vi "Parse Data to Clusters.vi"(8 "year":i32=1970, 9 "month":i32=1, 10 "day of month":i32=1, 11 "body Text":string) -> (3 "Result Data Array":T1[](array[typedef]))   [LabVIEW 2012]
uses:
  TypeDef/WeatherData.ctl
panel:
  out "Cleaned Text":string
  in  "Col Hedders":string[](array[string])
  out "Body Data":string[][](array[string])
  # "Time"
  # "Float"
  # "Float"
  # "Int"
  # "Float"
  # "Float"
  # "VARCHAR(10)"
  # "Float"
  # "Float"
  # "Float"
  # "VARCHAR(45)"
  # "VARCHAR(45)"
  # "INT"
  # "Date time"
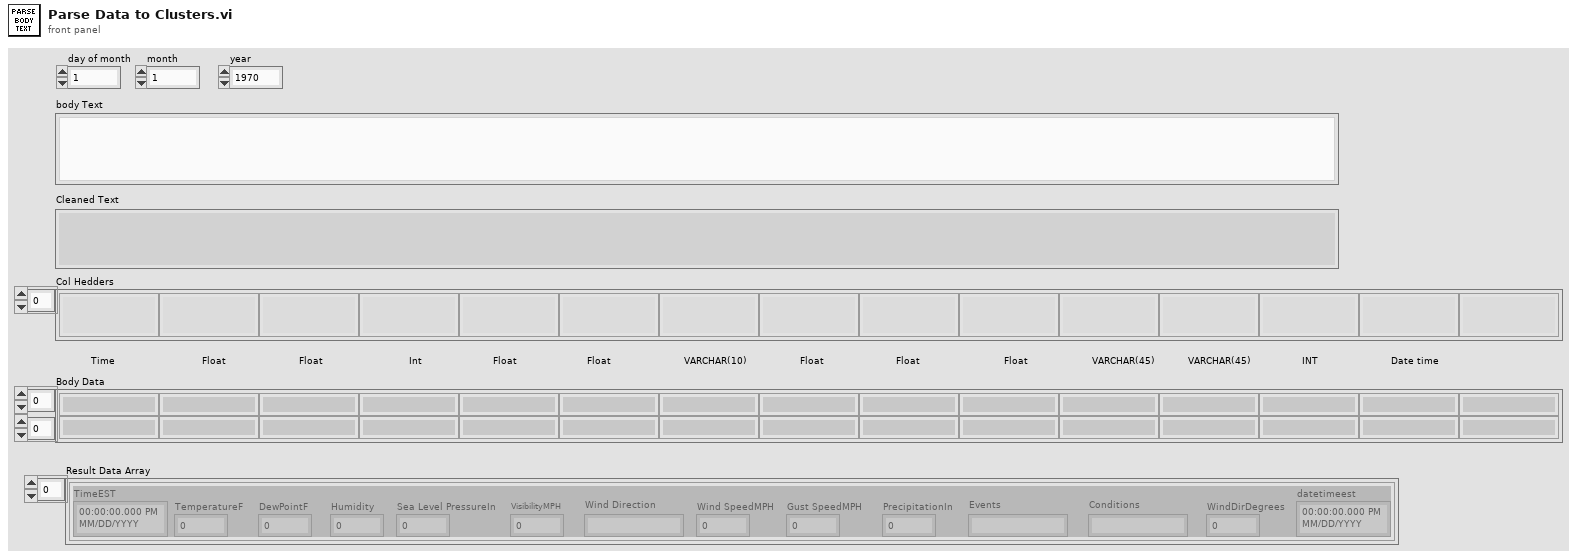
[diagram p1: front panel]
types:
  T1 = typedef "WeatherData.ctl" = cluster{"TimeEST":timestamp, "TemperatureF":dbl, "DewPointF":dbl, "Humidity":i32, "Sea Level PressureIn":dbl, "VisibilityMPH":dbl, "Wind Direction":string, "Wind SpeedMPH":dbl, "Gust SpeedMPH":dbl, "PrecipitationIn":dbl, "Events":string, "Conditions":string, "WindDirDegrees":i32, "datetimeest":timestamp}
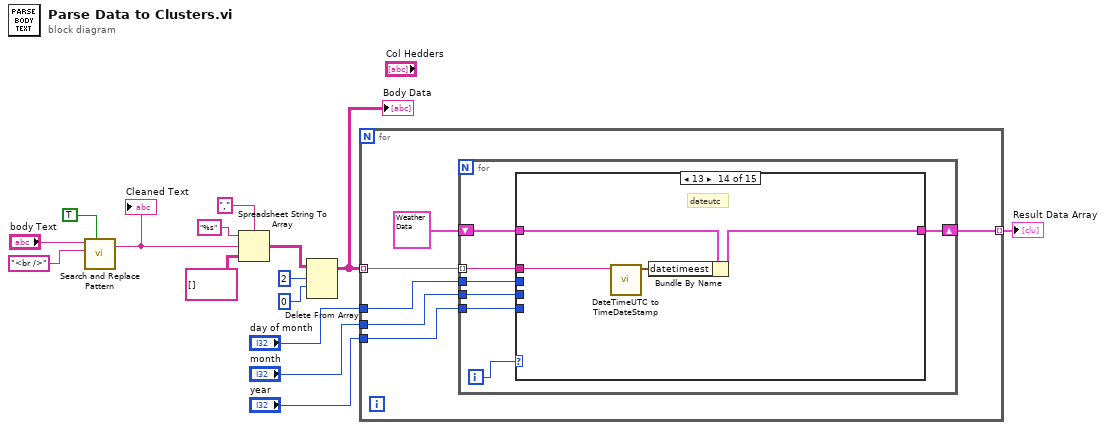
[diagram p0: block diagram]
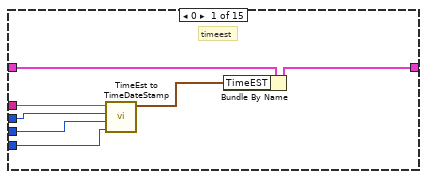
[diagram p2: hidden frame]
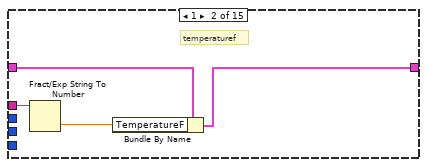
[diagram p3: hidden frame]
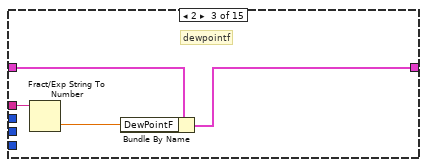
[diagram p4: hidden frame]
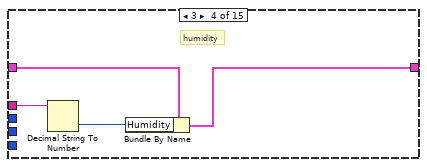
[diagram p5: hidden frame]
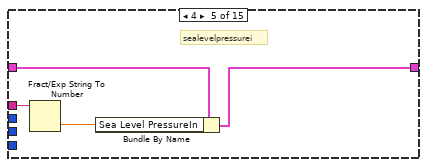
[diagram p6: hidden frame]
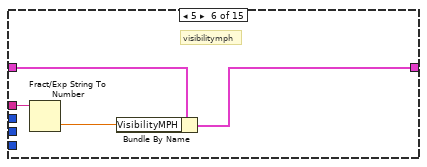
[diagram p7: hidden frame]
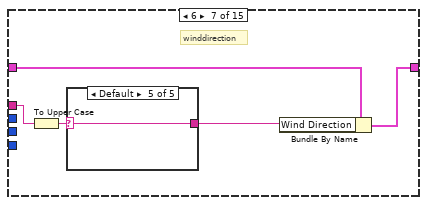
[diagram p8: hidden frame]
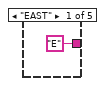
[diagram p9: hidden frame]
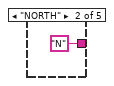
[diagram p10: hidden frame]
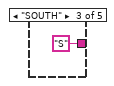
[diagram p11: hidden frame]
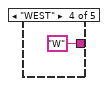
[diagram p12: hidden frame]
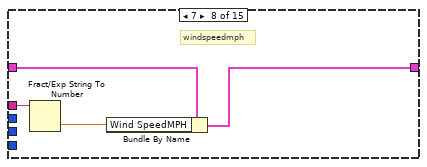
[diagram p13: hidden frame]
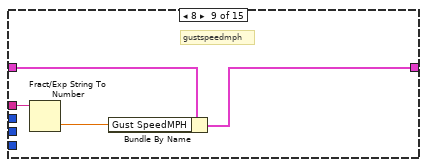
[diagram p14: hidden frame]
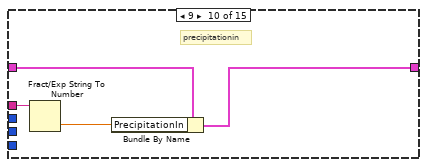
[diagram p15: hidden frame]
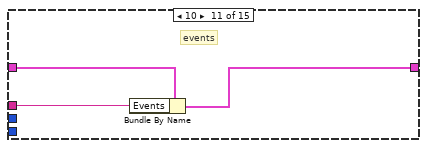
[diagram p16: hidden frame]
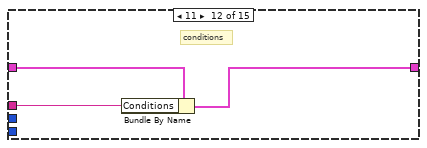
[diagram p17: hidden frame]
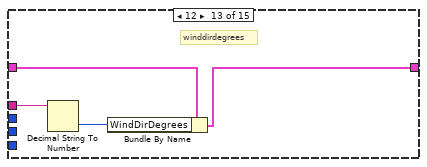
[diagram p18: hidden frame]
diagram:
  n1 = call <vilib>:"Search and Replace Pattern.vi"("string"="body Text", "regular expression (\"\")"="<br />" ("regular expression (\"\")"), "replace all? (F)"=TRUE) -> ("result string"=w6:string)  [unwired: 2 in, 1 out]
  "Cleaned Text" <- w6
  n2 = Spreadsheet String To Array(delimiter (Tab)=",", format string="%s", spreadsheet string=w6, array type (2D Dbl)=string[][] []) -> (array=w12:string[][])
  n3 = Delete From Array(array=w12, length=2, index (row)=0) -> (array with subset deleted=w9:string[][])  [unwired: 1 in, 1 out]
  "Body Data" <- w9
  n4 = for {
    tunnel: w9 -> [w20] mode=indexing
    tunnel: [w19] -> w8 mode=indexing
    tunnel: "day of month" -> [w18]
    tunnel: "month" -> [w17]
    tunnel: "year" -> [w16]
    n5 = for {
      tunnel: w20 -> [w27] mode=indexing
      shift-right: [w25] -> w19
      shift-left: T1 {"TimeEST"=timestamp(0 s since 1904-01-01), "TemperatureF"=0.0, "DewPointF"=0.0, "Humidity"=0, "Sea Level PressureIn"=0.0, "VisibilityMPH"=0.0, "Wind Direction"="", "Wind SpeedMPH"=0.0, "Gust SpeedMPH"=0.0, "PrecipitationIn"=0.0, "Events"="", "Conditions"="", "WindDirDegrees"=0, "datetimeest"=timestamp(0 s since 1904-01-01)} ("weatherdata") -> [w26]
      tunnel: w18 -> [w24]
      tunnel: w17 -> [w23]
      tunnel: w16 -> [w22]
      i -> [w28]
      n6 = case shown="13" w28 {
        tunnel: w27 -> [w33 w39 w43 w45 w51 w55 w58 w69 w73 w77 w78 w81 w85 w89 _]
        tunnel: w26 -> [w35 w37 w41 w47 w49 w53 w60 w67 w71 w75 w80 w83 w87 w91 w92]
        tunnel: [w34 w36 w40 w46 w48 w52 w59 w66 w70 w74 w79 w82 w86 w90 w92] -> w25
        tunnel: w24 -> [w31 _ _ _ _ _ _ _ _ _ _ _ _ _ _]
        tunnel: w23 -> [w30 _ _ _ _ _ _ _ _ _ _ _ _ _ _]
        tunnel: w22 -> [w29 _ _ _ _ _ _ _ _ _ _ _ _ _ _]
        frame 0 {
          # "timeest"
          n7 = call "TimeEst to TimeDateStamp.vi"("year"=w29, "month"=w30, "day of month"=w31, "Time String"=w33) -> ("time stamp"=w32:timestamp)  [unwired: 7 in]
          n8 = Bundle By Name(cluster=w35, "TimeEST"=w32) -> (w34:T1)
        }
        frame 1 {
          # "temperaturef"
          n9 = Fract/Exp String To Number(string=w39) -> (number=w38:dbl)  [unwired: 3 in, 1 out]
          n10 = Bundle By Name(cluster=w37, "TemperatureF"=w38) -> (w36:T1)
        }
        frame 2 {
          # "dewpointf"
          n11 = Fract/Exp String To Number(string=w43) -> (number=w42:dbl)  [unwired: 3 in, 1 out]
          n12 = Bundle By Name(cluster=w41, "DewPointF"=w42) -> (w40:T1)
        }
        frame 3 {
          # "humidity"
          n13 = Decimal String To Number(string=w45) -> (number=w44:i32)  [unwired: 2 in, 1 out]
          n14 = Bundle By Name(cluster=w47, "Humidity"=w44) -> (w46:T1)
        }
        frame 4 {
          # "sealevelpressurei"
          n15 = Fract/Exp String To Number(string=w51) -> (number=w50:dbl)  [unwired: 3 in, 1 out]
          n16 = Bundle By Name(cluster=w49, "Sea Level PressureIn"=w50) -> (w48:T1)
        }
        frame 5 {
          # "visibilitymph"
          n17 = Fract/Exp String To Number(string=w55) -> (number=w54:dbl)  [unwired: 3 in, 1 out]
          n18 = Bundle By Name(cluster=w53, "VisibilityMPH"=w54) -> (w52:T1)
        }
        frame 6 {
          # "winddirection"
          n19 = To Upper Case(1:w58) -> (0:w56:string)
          n20 = case shown="Default" w56 {
            selector: w56 -> [_ _ _ _ w65]
            tunnel: ["E" "N" "S" "W" w65] -> w57
            frame "EAST" {
            }
            frame "NORTH" {
            }
            frame "SOUTH" {
            }
            frame "WEST" {
            }
            frame Default {
            }
          }
          n21 = Bundle By Name(cluster=w60, "Wind Direction"=w57) -> (w59:T1)
        }
        frame 7 {
          # "windspeedmph"
          n22 = Fract/Exp String To Number(string=w69) -> (number=w68:dbl)  [unwired: 3 in, 1 out]
          n23 = Bundle By Name(cluster=w67, "Wind SpeedMPH"=w68) -> (w66:T1)
        }
        frame 8 {
          # "gustspeedmph"
          n24 = Fract/Exp String To Number(string=w73) -> (number=w72:dbl)  [unwired: 3 in, 1 out]
          n25 = Bundle By Name(cluster=w71, "Gust SpeedMPH"=w72) -> (w70:T1)
        }
        frame 9 {
          # "precipitationin"
          n26 = Fract/Exp String To Number(string=w77) -> (number=w76:dbl)  [unwired: 3 in, 1 out]
          n27 = Bundle By Name(cluster=w75, "PrecipitationIn"=w76) -> (w74:T1)
        }
        frame 10 {
          # "events"
          n28 = Bundle By Name(cluster=w80, "Events"=w78) -> (w79:T1)
        }
        frame 11 {
          # "conditions"
          n29 = Bundle By Name(cluster=w83, "Conditions"=w81) -> (w82:T1)
        }
        frame 12 {
          # "winddirdegrees"
          n30 = Decimal String To Number(string=w85) -> (number=w84:i32)  [unwired: 2 in, 1 out]
          n31 = Bundle By Name(cluster=w87, "WindDirDegrees"=w84) -> (w86:T1)
        }
        frame 13 {
          # "dateutc"
          n32 = call "DateTimeUTC to TimeDateStamp.vi"("Time String"=w89) -> ("time stamp"=w88:timestamp)  [unwired: 10 in]
          n33 = Bundle By Name(cluster=w91, "datetimeest"=w88) -> (w90:T1)
        }
        frame Default {
        }
      }
    }
  }
  "Result Data Array" <- w8
